vi "File_Build Valid Paths.vi"(7 "Run Data":T1={"Target Folder"=path "", "Menu Folder"=path "", "Active Folder"=path "", "Config"={"Main"={"Menu Folder"="", "Re-Create Menu Folder?"=FALSE, "Allow mnu replace?"=FALSE, "Relative Link Target"=""}, "File Filter"={"Exclude Prefixes"=[], "Ignore Names"=[], "Include Extensions"=[], "Exclude Postfixes"=[]}, "Folder Filter"={"Exclude Prefixes"=[], "Ignore Names"=[]}, "File Name Edit"={"Pre Split String"="", "Post Split String"="", "Deletion Strings"=[]}, "Folder Name Edit"={"Pre Split String"="", "Post Split String"="", "Deletion Strings"=[]}, "Folder Icon Map"={}, "Default Palette Data"={"Display Name Override"="", "View Format"=2, "Palette Width"=0, "Help Tag"="", "Help File Path"=path "", "Palette Description"=""}, "Default File Data"={"Display Name Override"="", "Place VI Contents?"=FALSE}, "Palette Override map"={}, "File Override map"={}}} {"Config"."Default Palette Data"."View Format" items=["Icons", "Text", "Icons and Text"]}, 8 "error in (no error)":errorcluster, 10 "File names":string[](array[string]), 11 "Active Path":path) -> (0 "error out":errorcluster, 3 "Valid File Paths":path[](array[path]))   [LabVIEW 2019, in "AutoMenuCreator.lvlib"]
uses:
  AutoMenuCreator.lvlib
  Ctl/Ctl_Run Data.ctl
  Ctl/Ctl_Config.ctl
  Ctl/Ctl_Config_Main.ctl
  Ctl/Ctl_Config_File Filter.ctl
  Ctl/Ctl_Config_Folder Filter.ctl
  Ctl/Ctl_Config_Name Edit.ctl
  Ctl/Ctl_Config_Folder Icon Map.ctl
  Ctl/Ctl_Config_Palette Data.ctl
  <vilib>/Palette API/Palette Menu/Public Type Define/View Format.ctl
  Ctl/Ctl_Config_File Data.ctl
  <vilib>/Palette API/Palette Menu/Palette Menu.lvlib
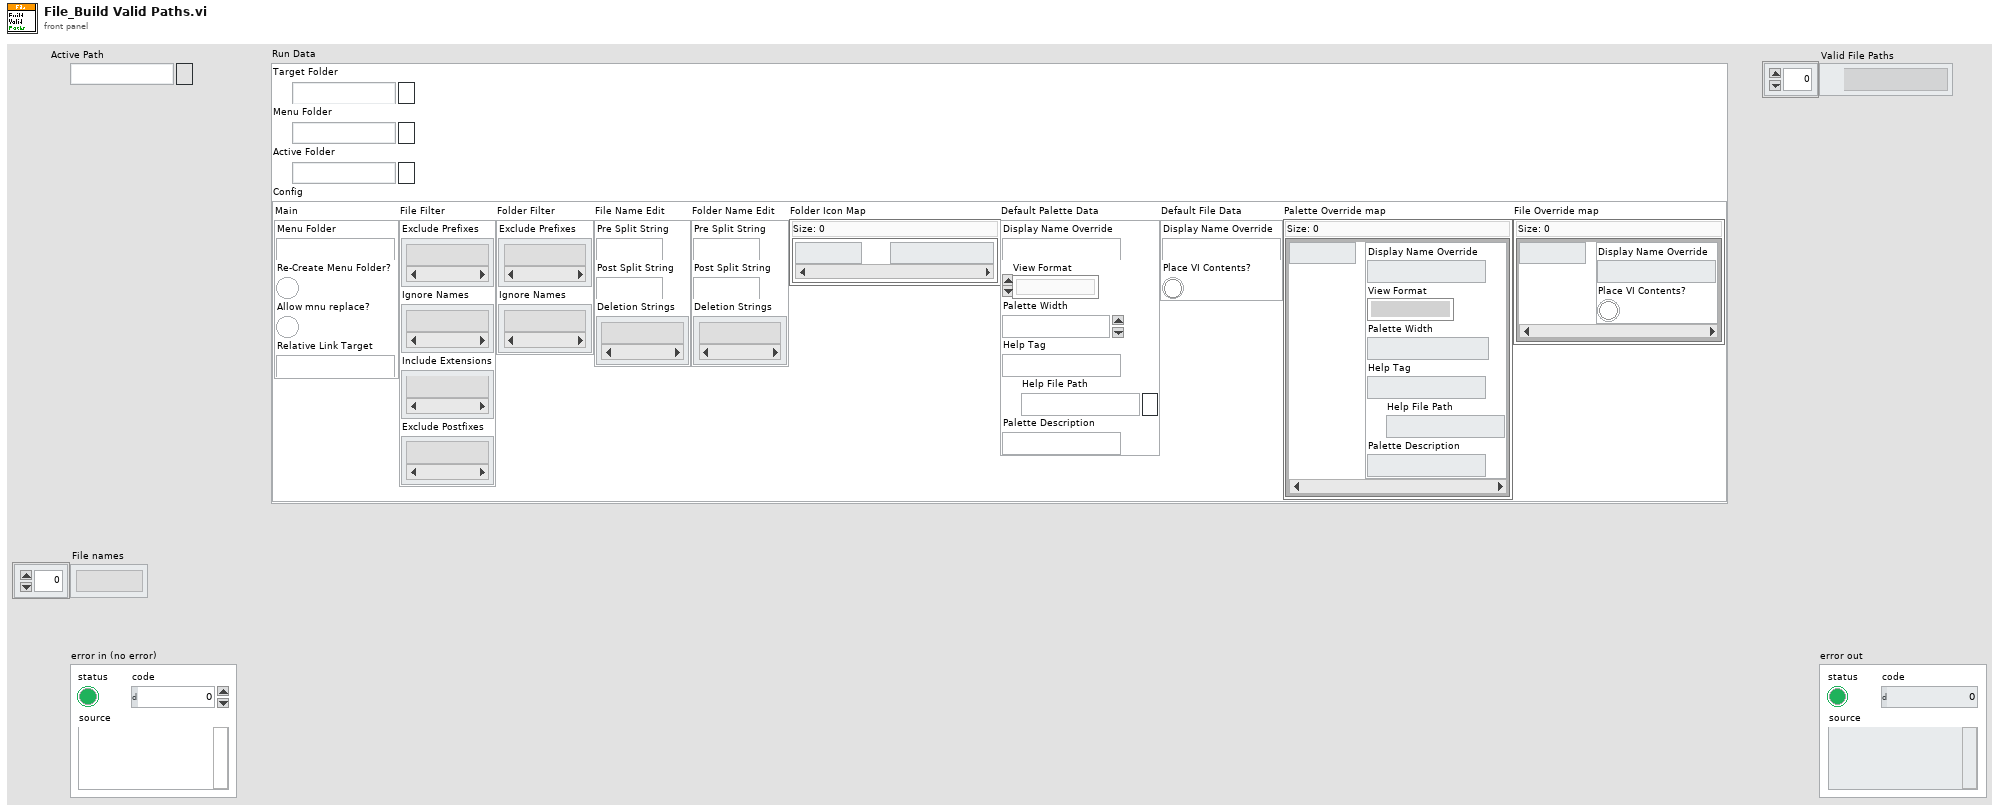
[diagram p1: front panel]
types:
  T1 = typedef "AutoMenuCreator.lvlib/Ctl_Run Data.ctl" = cluster{"Target Folder":path, "Menu Folder":path, "Active Folder":path, "Config":T2}
  T2 = typedef "AutoMenuCreator.lvlib/Ctl_Config.ctl" = cluster{"Main":T3, "File Filter":T4, "Folder Filter":T5, "File Name Edit":T6, "Folder Name Edit":T6, "Folder Icon Map":T7, "Default Palette Data":T8, "Default File Data":T10, "Palette Override map":map{string, T8}, "File Override map":map{string, T10}}
  T3 = typedef "AutoMenuCreator.lvlib/Ctl_Config_Main.ctl" = cluster{"Menu Folder":string, "Re-Create Menu Folder?":bool, "Allow mnu replace?":bool, "Relative Link Target":string}
  T4 = typedef "AutoMenuCreator.lvlib/Ctl_Config_File Filter.ctl" = cluster{"Exclude Prefixes":string[], "Ignore Names":string[], "Include Extensions":string[], "Exclude Postfixes":string[]}
  T5 = typedef "AutoMenuCreator.lvlib/Ctl_Config_Folder Filter.ctl" = cluster{"Exclude Prefixes":string[], "Ignore Names":string[]}
  T6 = typedef "AutoMenuCreator.lvlib/Ctl_Config_Name Edit.ctl" = cluster{"Pre Split String":string, "Post Split String":string, "Deletion Strings":string[]}
  T7 = typedef "AutoMenuCreator.lvlib/Ctl_Config_Folder Icon Map.ctl" = map{string, path}
  T8 = typedef "AutoMenuCreator.lvlib/Ctl_Config_Palette Data.ctl" = cluster{"Display Name Override":string, "View Format":T9, "Palette Width":i16, "Help Tag":string, "Help File Path":path, "Palette Description":string}
  T9 = typedef "Palette Menu.lvlib/View Format.ctl" = u16
  T10 = typedef "AutoMenuCreator.lvlib/Ctl_Config_File Data.ctl" = cluster{"Display Name Override":string, "Place VI Contents?":bool}
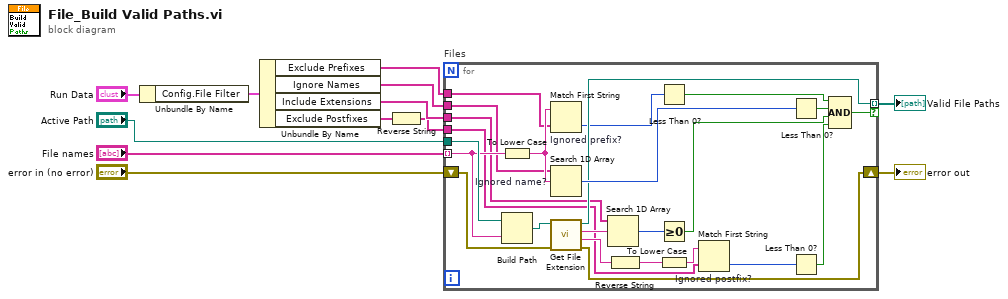
[diagram p0: block diagram]
diagram:
  n1 = Unbundle By Name("Run Data") -> ("Config.File Filter"=w1:T4)
  n2 = Unbundle By Name(w1) -> ("Exclude Prefixes"=w7:string[], "Ignore Names"=w6:string[], "Include Extensions"=w5:string[], "Exclude Postfixes"=w4:string[])
  n3 = Reverse String(1:w4) -> (0:w3:string[])
  n4 = for "Files" {
    tunnel: "File names" -> [w32] mode=indexing
    tunnel: [w27] -> w10 mode=indexing if=w34
    tunnel: "Active Path" -> [w33]
    shift-right: [w25] -> w11
    shift-left: "error in (no error)" -> [w26]
    tunnel: w7 -> [w16]
    tunnel: w6 -> [w15]
    tunnel: w5 -> [w14]
    tunnel: w3 -> [w13]
    n5 = To Lower Case(string=w32) -> (all lower case string=w22:string)
    n6 = Build Path(base path=w33, name or relative path=w32) -> (appended path=w31:path)
    n7 = Match First String "Ignored prefix?"(2:w16, 3:w22) -> (0:w24:i32)  [unwired: 1 out]
    n8 = Search 1D Array "Ignored name?"(1D array=w15, element=w22) -> (index of element=w36:i32)  [unwired: 1 in]
    n9 = call <vilib>:"Get File Extension.vi"("error in (no error)"=w26, "file"=w31) -> ("error out"=w25:errorcluster, "filename without extension"=w21:string, "lowercase file extension"=w30:string, "dup file"=w27:path)  [unwired: 5 in, 1 out]
    n10 = Search 1D Array(1D array=w14, element=w30) -> (index of element=w29:i32)  [unwired: 1 in]
    n11 = Reverse String(1:w21) -> (0:w20:string)
    n12 = Less Than 0?(x=w24) -> (x < 0?=w23:bool)
    n13 = Greater Or Equal To 0?(x=w29) -> (x >= 0?=w28:bool)
    n14 = To Lower Case(string=w20) -> (all lower case string=w19:string)
    n15 = Match First String "Ignored postfix?"(2:w13, 3:w19) -> (0:w18:i32)  [unwired: 1 out]
    n16 = Less Than 0?(x=w36) -> (x < 0?=w35:bool)
    n17 = Less Than 0?(x=w18) -> (x < 0?=w17:bool)
    n18 = Compound Arithmetic op=AND(w23, w35, w28, w17) -> (w34:bool)
  }
  "error out" <- w11
  "Valid File Paths" <- w10
